vi "Divider2.vi"() -> (8 "Divider2":refnum<class "Divider2.lvclass">)   [LabVIEW 2017, in "Divider2.lvclass"]
uses:
  Divider2.lvclass
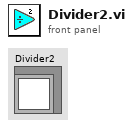
[diagram p1: front panel]
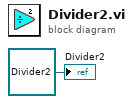
[diagram p0: block diagram]
diagram:
  "Divider2" <- refnum<class "Divider2.lvclass"> refnum ("Divider2.lvclass")
